vi "Pockels Cal-Spline interpolate objectives cal.vi"(11 "Pockels Cal table":string[][](array[string])=[["0", "0", "0", "0"], ["0.1", "2.8", "", ""], ["0.2", "9.8", "6.86", ""], ["0.3", "21.4", "", ""], ["0.4", "37.1", "25.97", "37.1"], ["0.5", "56.1", "", ""], ["0.6", "77.7", "54.39", ""], ["0.7", "101", "", ""], ["0.8", "125", "87.5", "125"], ["0.9", "148", "", ""], ["1", "169", "118.3", ""], ["1.1", "188", "", ""], ["1.2", "204", "142.8", "204"], ["1.3", "215", "", ""], ["1.4", "222", "155.4", ""], ["1.5", "225", "", ""], ["1.6", "222", "155.4", "222"], ["1.7", "214", "", ""], ["1.8", "202", "141.4", ""], ["1.9", "187", "", ""], ["2", "152", "106.4", "152"]]) -> (3 "Spline-Interpolated":dbl[][](array[numeric]))   [LabVIEW 2020]
uses:
  <userlib>/_OpenG.lib/array/array.llb/Search 1D Array (String)__ogtk.vi
  <userlib>/_OpenG.lib/array/array.llb/Delete Elements from 1D Array (DBL)__ogtk.vi
  <vilib>/gmath/NI_Gmath.lvlib
panel:
  in  "Pockels Cal table 2":string[][](array[string])=[["0", "0", "0", "0"], ["0.1", "2.8", "1.96", ""], ["0.2", "9.8", "6.86", ""], ["0.3", "21.4", "14.98", ""], ["0.4", "37.1", "25.97", "37.1"], ["0.5", "56.1", "39.27", ""], ["0.6", "77.7", "54.39", ""], ["0.7", "101", "70.7", ""], ["0.8", "125", "87.5", "125"], ["0.9", "148", "103.6", ""], ["1", "169", "118.3", ""], ["1.1", "188", "131.6", ""], ["1.2", "204", "142.8", "204"], ["1.3", "215", "150.5", ""], ["1.4", "222", "155.4", ""], ["1.5", "225", "157.5", ""], ["1.6", "222", "155.4", "222"], ["1.7", "214", "149.8", ""], ["1.8", "202", "141.4", ""], ["1.9", "187", "130.9", ""], ["2", "152", "106.4", "152"]]
  out "array w/ subset deleted":dbl[](array[numeric]) format="%.2f"
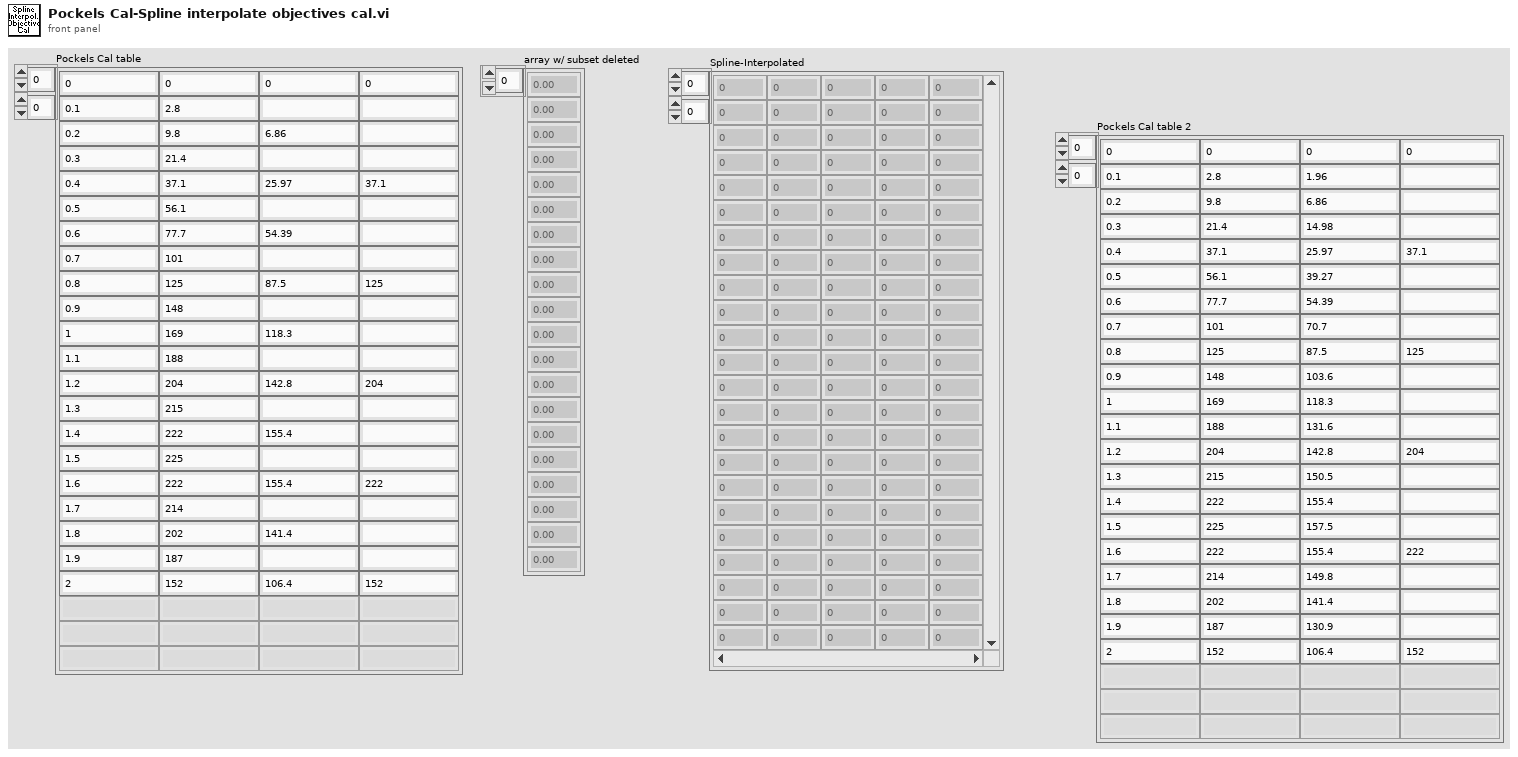
[diagram p1: front panel]
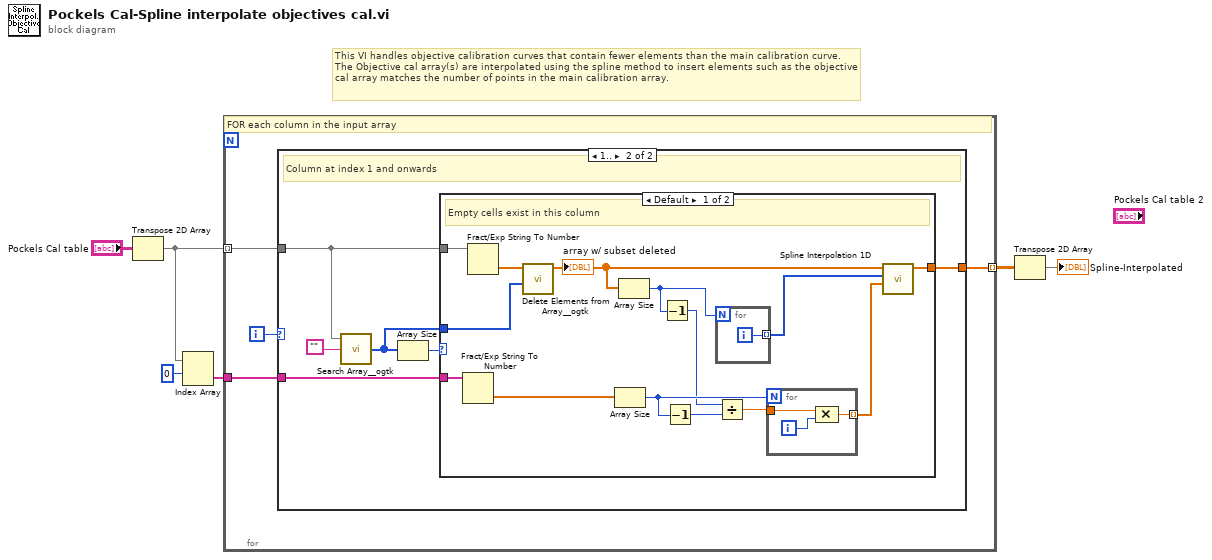
[diagram p0: block diagram]
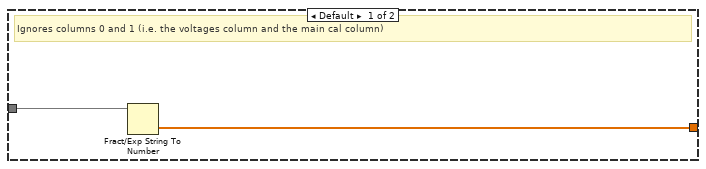
[diagram p2: hidden frame]
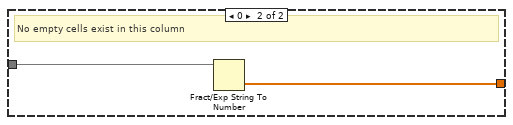
[diagram p3: hidden frame]
diagram:
  # "This VI handles objective calibration curves that contain fewer elements than the main calibration curve. The Objective cal array(s) are interpolated using the spline method to insert elements such as the objective cal array matches the number of points in the main calibration array."
  n1 = Transpose 2D Array(2D array="Pockels Cal table") -> (transposed array=w4:string[][])
  n2 = Index Array(array=w4, index (row)=0) -> (element=w2:string[])  [unwired: 1 in]
  n3 = for {
    tunnel: w4 -> [w10] mode=indexing
    tunnel: [w9] -> w5 mode=indexing
    tunnel: w2 -> [w8]
    i -> [w7]
    # "FOR each column in the input array"
    n4 = case shown="1.." w7 {
      tunnel: w10 -> [w12 w16]
      tunnel: [w11 w15] -> w9
      tunnel: w8 -> [_ w13]
      frame Default {
        # "Ignores columns 0 and 1 (i.e. the voltages column and the main cal column)"
        n5 = Fract/Exp String To Number(string=w12) -> (number=w11:dbl[])  [unwired: 3 in, 1 out]
      }
      frame 1.. {
        # "Column at index 1 and onwards"
        n6 = call-poly <userlib>:"Search Array__ogtk.vi"("Array"=w16, "Element Data"="" ("element")) -> ("Indices of Elements"=w14:i32[])  [unwired: 7 in]
        n7 = Array Size(array=w14) -> (size(s)=w17:i32)
        n8 = case shown="Default" w17 {
          tunnel: w16 -> [w32 w38]
          tunnel: [w19 w37] -> w15
          tunnel: w14 -> [w31 _]
          tunnel: w13 -> [w30 _]
          frame Default {
            # "Empty cells exist in this column"
            n9 = Fract/Exp String To Number(string=w30) -> (number=w27:dbl[])  [unwired: 3 in, 1 out]
            n10 = Fract/Exp String To Number(string=w32) -> (number=w29:dbl[])  [unwired: 3 in, 1 out]
            n11 = call-poly <userlib>:"Delete Elements from Array__ogtk.vi"("indices"=w31, "array"=w29) -> ("array w/ subset deleted"=w20:dbl[])  [unwired: 8 in, 1 out]
            "array w/ subset deleted" <- w20
            n12 = Array Size(array=w27) -> (size(s)=w26:i32)
            n13 = Array Size(array=w20) -> (size(s)=w23:i32)
            n14 = Decrement(x=w23) -> (x-1=w21:i32)
            n15 = Decrement(x=w26) -> (x-1=w22:i32)
            n16 = for {
              N: w23 -> [_]
              tunnel: [w36] -> w28 mode=indexing
              i -> [w36]
            }
            n17 = Divide(x=w21, y=w22) -> (x/y=w24:dbl)
            n18 = for {
              N: w26 -> [_]
              tunnel: [w35] -> w25 mode=indexing
              tunnel: w24 -> [w34]
              i -> [w33]
              n19 = Compound Arithmetic op=MULTIPLY(w34, w33) -> (w35:dbl)
            }
            n20 = call <vilib>:"Spline Interpolation 1D.vi"("xi"=w25, "X"=w28, "Y"=w20) -> ("yi"=w19:dbl[])  [unwired: 6 in, 2 out]
          }
          frame 0 {
            # "No empty cells exist in this column"
            n21 = Fract/Exp String To Number(string=w38) -> (number=w37:dbl[])  [unwired: 3 in, 1 out]
          }
        }
      }
    }
  }
  n22 = Transpose 2D Array(2D array=w5) -> (transposed array=→"Spline-Interpolated":dbl[][])
